vi "Set Blending.vi"(4 "Source":T3(ring)=enum."Source Alpha", 6 "Destination":T2(ring)=enum."One Minus Source Alpha", 8 "error in (no error)":errorcluster, 9 "Bin":T1(ring), 10 "Mode":enum16{"Inherit Value", "Off", "On"}(ring), 11 "Scene Object In":refnum<vi>) -> (0 "error out":errorcluster, 3 "Scene Object Out":refnum<vi>)   [LabVIEW 2020, in "NI_3D Picture Control.lvlib"]
doc: "Blends fragment color outputs with destination colors for texturing 3D objects."
uses:
  <vilib>/picture/3D Picture Control/NI_3D Picture Control.lvlib
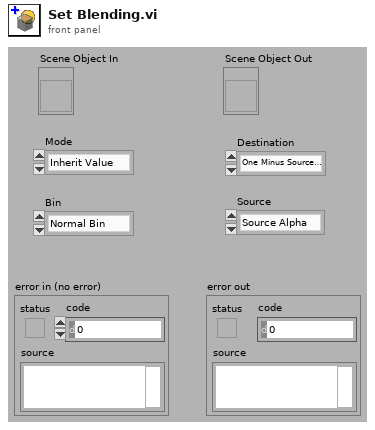
[diagram p1: front panel]
types:
  T1 = enum16{"Normal Bin", "Opaque Bin", "Transparent Bin"}
  T2 = enum16{"Zero", "One", "Source Color", "One Minus Source Color", "Source Alpha", "One Minus Source Alpha", "Destination Alpha", "One Minus Destination Alpha"}
  T3 = enum16{"Zero", "One", "Destination Color", "One Minus Destination Color", "Source Alpha", "One Minus Source Alpha", "Destination Alpha", "One Minus Destination Alpha", "Source Alpha Saturate"}
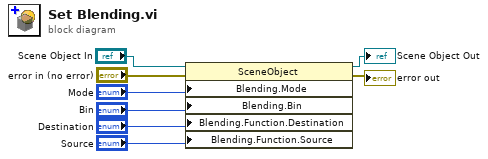
[diagram p0: block diagram]
diagram:
  n1 = property class="SceneObject"(reference="Scene Object In", error in="error in (no error)", "Blending.Mode"="Mode", "Blending.Bin"="Bin", "Blending.Function.Destination"="Destination", "Blending.Function.Source"="Source") -> (reference out=→"Scene Object Out":refnum<vi>, error out=→"error out":errorcluster)
